vi "Untitled 1.vi"() -> ()   [LabVIEW 2023]
uses:
  <vilib>/userDefined/High Color/nirio_resource_hc.ctl
  <vilib>/FPGAPlugInAG/cRIO-9030/niLvFpga_Open_cRIO-9030.vi
  <vilib>/rvi/interface/common/dynamic/niFpgaDynamicAddResources.vi
  <vilib>/FPGAPlugInAG/Dynamic/niLvFpga_Reset_Dynamic.vi
  <vilib>/FPGAPlugInAG/Dynamic/niLvFpga_Run_Dynamic.vi
  <vilib>/Utility/error.llb/Error Cluster From Error Code.vi
  <vilib>/rvi/errors/niLvFpgaAdjustHostInterfaceError.vi
  <vilib>/FPGAPlugInAG/Dynamic/niLvFpga_Close_Dynamic.vi
  <vilib>/rvi/interface/nirviOpenFPGA/nirviOpenFPGA.xnode
  pbl_FPGATarget_FPGATEST_QgjEpZd9ZEg.lvbitx
  <vilib>/rvi/interface/nirviMethod/nirviMethod.xnode
  <vilib>/rvi/interface/nirviReadWriteControl/nirviReadWriteControl.xnode
  <vilib>/rvi/interface/nirviCloseFPGA/nirviCloseFPGA.xnode
  NiFpgaLv.dll
  <vilib>/rvi/interface/Simulation/niFpgaSimulationCallBeginRW.vi
panel:
  in  "Duty Cycle 0-100":sgl
  in  "Numeric":i32
  in  "Digital 2 ON/OFF":bool
  in  "stop":bool
  in  "Digital 1 ON/OFF":bool
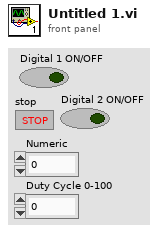
[diagram p1: front panel]
types:
  T1 = typedef "nirio_resource_hc.ctl" = tag
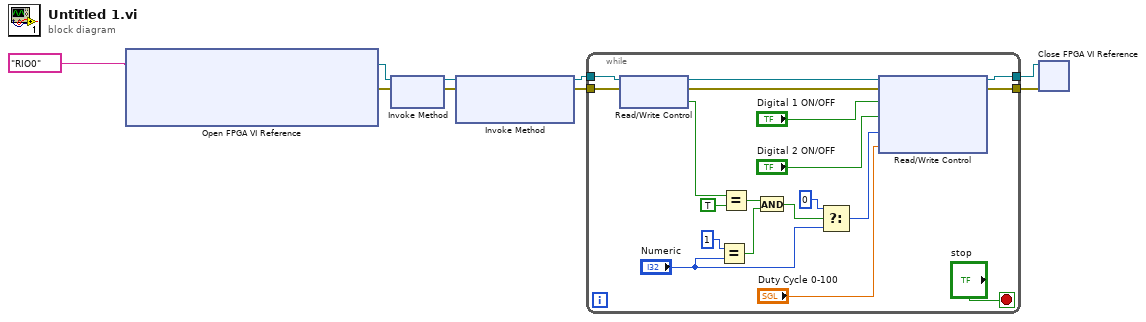
[diagram p0: block diagram]
diagram:
  n1 = xnode "Open FPGA VI Reference"("resource name"=T1 "RIO0") -> ("FPGA VI Reference Out"=w9:refnum<k20>, "error out"=w8:errorcluster)  [unwired: 1 in]
  n2 = xnode "Invoke Method"("FPGA VI Reference In"=w9, "error in"=w8) -> ("FPGA VI Reference Out"=w6:refnum<k20>, "error out"=w7:errorcluster)
  n3 = xnode "Invoke Method"("FPGA VI Reference In"=w6, "error in"=w7) -> ("FPGA VI Reference Out"=w4:refnum<k20>, "error out"=w5:errorcluster)  [unwired: 1 in]
  n4 = while {
    tunnel: w5 -> [w24]
    tunnel: w4 -> [w23]
    tunnel: [w11] -> w3
    tunnel: [w10] -> w2
    stop <- "stop" stop-if-true
    n5 = xnode "Read/Write Control"("FPGA VI Reference In"=w23, "error in"=w24) -> ("FPGA VI Reference Out"=w22:refnum<k20>, "error out"=w21:errorcluster, "Running?"=w20:bool)
    n6 = Equal?(x=1, y="Numeric") -> (x = y?=w17:bool)
    n7 = Equal?(x=w20, y=TRUE) -> (x = y?=w16:bool)
    n8 = And(x=w16, y=w17) -> (x .and. y?=w15:bool)
    n9 = Select(t=0, s=w15, f="Numeric") -> (s? t:f=w12:i32)
    n10 = xnode "Read/Write Control"("FPGA VI Reference In"=w22, "error in"=w21, "Digital 1 ON/OFF"="Digital 1 ON/OFF", "Digital 2 ON/OFF"="Digital 2 ON/OFF", "State PWM"=w12, "Duty Cycle 0-100"="Duty Cycle 0-100") -> ("FPGA VI Reference Out"=w10:refnum<k20>, "error out"=w11:errorcluster)
  }
  n11 = xnode "Close FPGA VI Reference"("FPGA VI Reference In"=w2, "error in"=w3) -> ()  [unwired: 1 out]
